vi "Turn To Angle.vi"(8 "Turn Angle Tolerance":dbl=2.0 format="%#_13g", 9 "output range":cluster{"output high":dbl, "output low":dbl}={"output high"=0.75, "output low"=-0.75}, 11 "Setpoint":dbl=143.0) -> (3 "Done?":bool=TRUE)   [LabVIEW 2016]
doc: "Turns the robot to a given gyro angle."
uses:
  Robot Values.vi
  <vilib>/addons/control/pid/pid.llb/PID (DBL).vi
  <vilib>/addons/control/pid/NI_PID_pid.lvlib
  <vilib>/ptbypt/NI_PtbyPt.lvlib
panel:
  out "Sensors.Gyro Angle":u16=143
  in  "Time Target (s)":dbl=0.15 format="%#_13g"
  out "Elapsed Time (s)":dbl=0.15655803680419922
  in  "PID gains":T1={"proportional gain (Kc)"=0.06, "integral time (Ti, min)"=0.0, "derivative time (Td, min)"=0.0} {"derivative time (Td, min)" format="%.3f"; "integral time (Ti, min)" format="%.3f"; "proportional gain (Kc)" format="%.3f"}
  # "Comp:\n.033\n0\n0"
  # "Practice:\n.07\n0\n0"
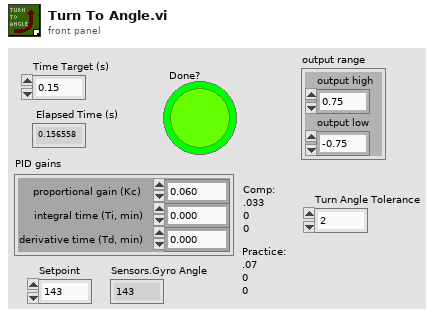
[diagram p1: front panel]
types:
  T1 = cluster{"proportional gain (Kc)":dbl, "integral time (Ti, min)":dbl, "derivative time (Td, min)":dbl}
  T2 = typedef "Robot Values.ctl" = cluster{"Robot Drive":cluster{"Left Motor Power":dbl, "Right Motor Power":dbl, "Left Encoder Value":dbl, "Right Encoder Value":dbl, "High Gear?":bool, "PTO?":bool}, "Sensors":cluster{"Gyro Angle":u16, "Recalibrate Gyro":bool, "Reset Gyro":bool, "Ultrasonic":dbl}, "Shooter":cluster{"Prep Wheels":bool, "Shoot":bool, "Left Shooter Wheel Speed":dbl, "Wheels Moving":bool, "Shooter Prepped":bool, "Shooter RPS SP":dbl, "Shooting?":bool, "Left Shooter Wheel Power":dbl, "Right Shooter Wheel Power":dbl, "Acquisition Conveyor Power":dbl, "Hopper Beater Bar Power":dbl, "Filtered Left Shooter Speed":dbl, "Acquisition Motor Power":dbl, "Joystick Add":dbl, "D-Pad Add":dbl, "Shooter Use PID?":bool}, "Robot States":cluster{"Drive mode":string, "Alliance":T3, "Position":T4}, "Gear":cluster{"Ejection Active":bool}}
  T3 = typedef "WPI_DriverStationAllianceInfo.ctl" = enum16{"Red", "Blue", "Invalid"}
  T4 = typedef "WPI_DriverStationPositionInfo.ctl" = enum16{"1", "2", "3"}
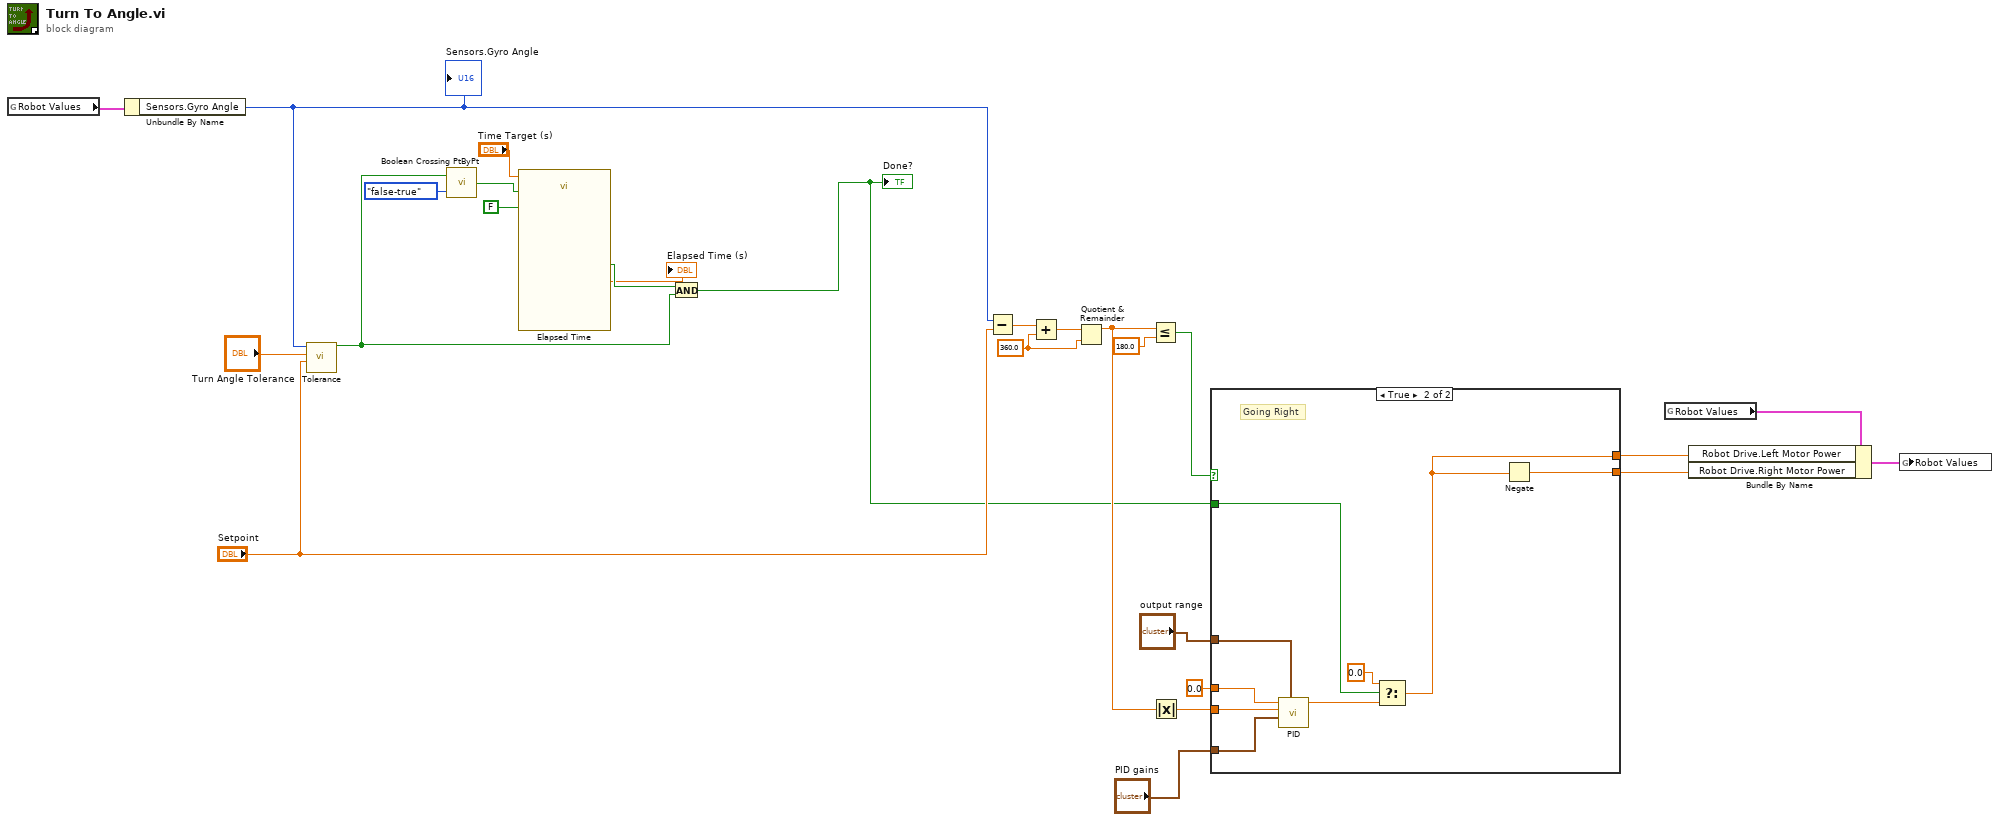
[diagram p0: block diagram]
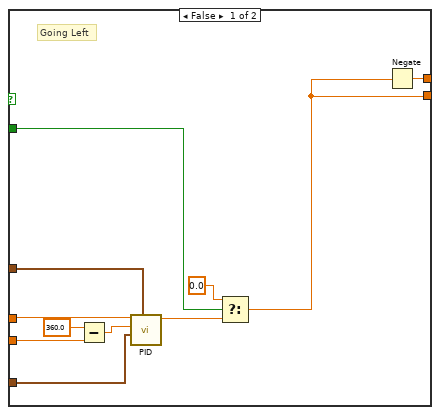
[diagram p2: hidden frame]
diagram:
  w23 = 360.0 ("y")
  n1 = global read "Robot Values.vi" "Robot Values"() -> (w26:T2)
  n2 = Unbundle By Name(w26) -> ("Sensors.Gyro Angle"=w11:u16)
  "Sensors.Gyro Angle" <- w11
  n3 = call "Tolerance.vi"("Setpoint"="Setpoint", "Tolerance"="Turn Angle Tolerance", "Current Value"=w11) -> ("In Range?"=w8:bool)  [unwired: 8 in]
  n4 = call <vilib>:"Boolean Crossing PtByPt.vi"("direction"=enum16{"either", "false-true", "true-false"}."false-true", "input"=w8) -> ("crossing"=w5:bool)  [unwired: 1 in]
  n5 = call "Elapsed Time"("Time Target (s)"="Time Target (s)", "Reset"=w5, "Auto Reset"=FALSE) -> ("Elapsed Time (s)"=→"Elapsed Time (s)":dbl, "Time has Elapsed"=w2:bool)  [unwired: 9 in, 6 out]
  n6 = And(x=w2, y=w8) -> (x .and. y?=w7:bool)
  "Done?" <- w7
  n7 = Subtract(x=w11, y="Setpoint") -> (x-y=w25:dbl)
  n8 = Add(x=w25, y=w23) -> (x+y=w24:dbl)
  n9 = Quotient & Remainder(x=w24, y=w23) -> (x-y*floor(x/y)=w14:dbl)  [unwired: 1 out]
  n10 = Less Or Equal?(x=w14, y=180.0) -> (x <= y?=w21:bool)
  n11 = Absolute Value(x=w14) -> (abs(x)=w12:dbl)
  n12 = case shown="True" w21 {
    tunnel: [w28 w40] -> w18
    tunnel: [w29 w39] -> w17
    tunnel: "PID gains" -> [w35 w46]
    tunnel: 0.0 ("setpoint") -> [w36 w45]
    tunnel: w12 -> [w34 w43]
    tunnel: "output range" -> [w37 w44]
    tunnel: w7 -> [w27 w38]
    frame False {
      # "Going Left"
      n13 = Subtract(x=360.0, y=w34) -> (x-y=w33:dbl)
      n14 = call-poly <vilib>:"PID.vi"("output range"=w37, "PID gains"=w35, "process variable"=w33, "setpoint"=w36) -> ("output"=w31:dbl)  [unwired: 6 in, 1 out]
      n15 = Select(t=0.0, s=w27, f=w31) -> (s? t:f=w29:dbl)
      n16 = Negate(x=w29) -> (-x=w28:dbl)
    }
    frame True {
      # "Going Right"
      n17 = call-poly <vilib>:"PID.vi"("output range"=w44, "PID gains"=w46, "process variable"=w43, "setpoint"=w45) -> ("output"=w42:dbl)  [unwired: 6 in, 1 out]
      n18 = Select(t=0.0, s=w38, f=w42) -> (s? t:f=w40:dbl)
      n19 = Negate(x=w40) -> (-x=w39:dbl)
    }
  }
  n20 = global read "Robot Values.vi" "Robot Values"() -> (w20:T2)
  n21 = Bundle By Name(cluster=w20, "Robot Drive.Left Motor Power"=w18, "Robot Drive.Right Motor Power"=w17) -> (w19:T2)
  n22 = global write "Robot Values.vi" "Robot Values"(w19) -> ()
